vi "terminate_scanners.vi"(8 "error in (no error)":errorcluster, 11 "DL090202ScanHead in":refnum<class "ScanHeadDL090202.lvclass">) -> (0 "error out":errorcluster, 3 "DL090202ScanHead out":refnum<class "ScanHeadDL090202.lvclass">)   [LabVIEW 2010, in "ScanHeadDL090202.lvclass"]
uses:
  ScanHeadDL090202.lvclass
  SignalWriter/GenericSignalWriter/GenericSignalWriter/GenericSignalWriter.lvclass
  common/classes/ErrorController/ErrorController/class_data.vi
  common/classes/ErrorController/ErrorController/ErrorController.lvclass
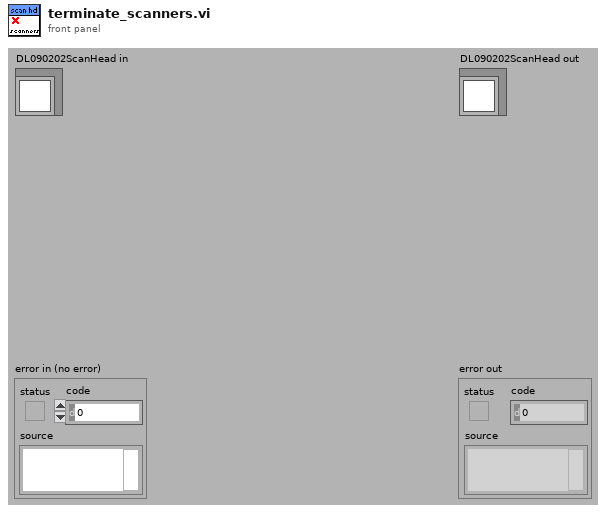
[diagram p1: front panel]
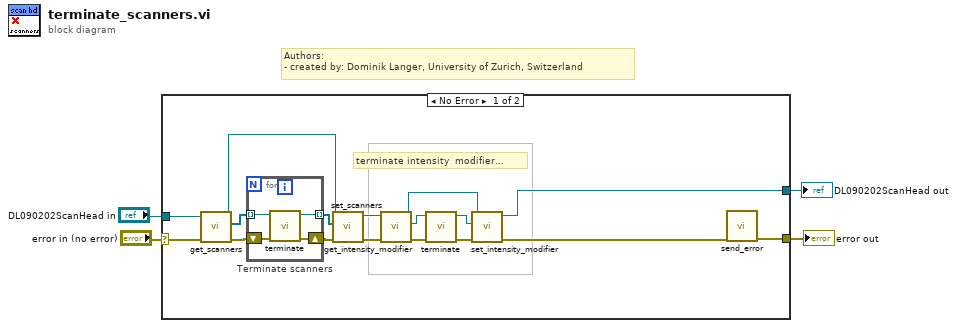
[diagram p0: block diagram]
diagram:
  # "Authors: \n- created by: Dominik Langer, University of Zurich, Switzerland"
  n1 = case shown="No Error" "error in (no error)" {
    selector: "error in (no error)" -> [w9 w27]
    tunnel: [w7 w27] -> w3
    tunnel: [w5 w26] -> w1
    tunnel: "DL090202ScanHead in" -> [w8 w26]
    frame No Error {
      # "terminate intensity  modifier..."
      n2 = call-dynamic "get_scanners.vi"("error in (no error)"=w9, "DL090202ScanHead.lvclass in"=w8) -> ("error out"=w10:errorcluster, "scanners"=w11:refnum<class "GenericSignalWriter.lvclass">[], "DL090202ScanHead.lvclass out"=w12:refnum<class "ScanHeadDL090202.lvclass">)  [unwired: 7 out]
      n3 = for "Terminate scanners" {
        shift-right: [w23] -> w14
        shift-left: w10 -> [w25]
        tunnel: [w24] -> w16 mode=indexing
        tunnel: w11 -> [w22] mode=indexing
        n4 = call-dynamic "terminate.vi"("error in (no error)"=w25, "GenericPlugin in"=w22) -> ("error out"=w23:errorcluster, "GenericPlugin out"=w24:refnum<class "GenericSignalWriter.lvclass">)  [unwired: 8 out]
      }
      n5 = call-dynamic "set_scanners.vi"("error in (no error)"=w14, "scanners"=w16, "DL090202ScanHead.lvclass in"=w12) -> ("error out"=w13:errorcluster, "DL090202ScanHead.lvclass out"=w17:refnum<class "ScanHeadDL090202.lvclass">)  [unwired: 7 out]
      n6 = call-dynamic "get_intensity_modifier.vi"("error in (no error)"=w13, "DL090202ScanHead.lvclass in"=w17) -> ("error out"=w15:errorcluster, "write signals"=w18:refnum<class "GenericSignalWriter.lvclass">, "DL090202ScanHead.lvclass out"=w21:refnum<class "ScanHeadDL090202.lvclass">)  [unwired: 7 out]
      n7 = call-dynamic "terminate.vi"("error in (no error)"=w15, "GenericPlugin in"=w18) -> ("error out"=w19:errorcluster, "GenericPlugin out"=w20:refnum<class "GenericSignalWriter.lvclass">)  [unwired: 8 out]
      n8 = call-dynamic "set_intensity_modifier.vi"("error in (no error)"=w19, "write signals"=w20, "DL090202ScanHead.lvclass in"=w21) -> ("error out"=w6:errorcluster, "DL090202ScanHead.lvclass out"=w5:refnum<class "ScanHeadDL090202.lvclass">)  [unwired: 7 out]
      n9 = call "send_error.vi"("error in (no error)"=w6) -> ("error out"=w7:errorcluster)  [unwired: 10 in]
    }
    frame Error {
    }
  }
  "error out" <- w3
  "DL090202ScanHead out" <- w1
